vi "Ancestor Classes.vi"(8 "error in (no error)":errorcluster, 11 "Section 2a in":refnum<class "Section 2a.lvclass">) -> (0 "error out":errorcluster, 1 "Ancestor Classes":string[](array[string]), 2 "Ancestor Class Pathes":path[](array[path]), 3 "Section 2a out":refnum<class "Section 2a.lvclass">)   [LabVIEW 2016, in "LVOOP Introduction.lvlib" / "Section 2a.lvclass"]
doc: "This VI returns array of all ancestor classes and their pathes."
uses:
  Section 2a.lvclass
  Section 2/Section 2.lvclass
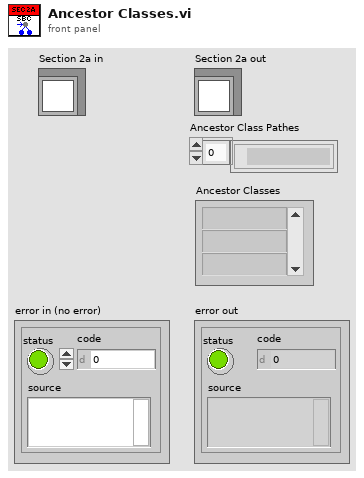
[diagram p1: front panel]
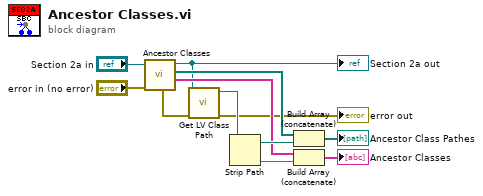
[diagram p0: block diagram]
diagram:
  n1 = call-parent "Ancestor Classes.vi"("error in (no error)"="error in (no error)", "Section 2 in"="Section 2a in") -> ("error out"=w10:errorcluster, "Ancestor Classes"=w7:string[], "Ancestor Class Pathes"=w8:path[], "Section 2 out"=w4:refnum<class "Section 2a.lvclass">)  [unwired: 6 in]
  "Section 2a out" <- w4
  n2 = call <vilib>:"Get LV Class Path.vi"("error in (no error)"=w10, "object"=w4) -> ("error out"=→"error out":errorcluster, "class path"=w9:path)  [unwired: 8 in]
  n3 = Strip Path(path=w9) -> (stripped path=w11:path, name=w12:string)
  n4 = Build Array (concatenate)(w8, w11) -> (→"Ancestor Class Pathes":path[])
  n5 = Build Array (concatenate)(w7, w12) -> (→"Ancestor Classes":string[])
